vi "SMBus Block Read.vi"(5 "PEC":u8, 6 "CommandCode":u8, 7 "SlaveAddr":u8, 9 "SMBUSIndex":i32, 10 "DevIndex":i32, 11 "DevType":i32) -> (1 "function return":i32, 2 "pByteCount":u8, 3 "pData":u8[](array[numeric]))   [LabVIEW 2010, in "ControlSMBus.lvlib"]
doc: "int WINAPI SMBus_BlockRead(int DevType,int DevIndex,int SMBUSIndex,unsigned char SlaveAddr,unsigned char CommandCode,unsigned char *pData,unsigned char *pByteCount,unsigned char PEC);"
uses:
  ControlSMBus.lvlib
  ControlSMBus/Ginkgo_Driver.dll
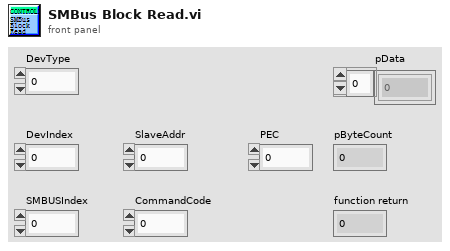
[diagram p1: front panel]
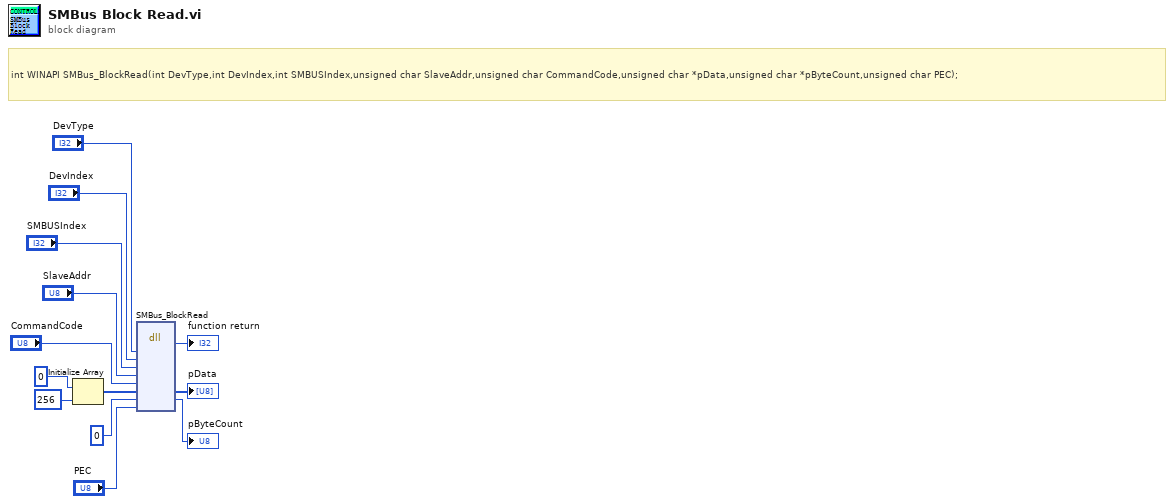
[diagram p0: block diagram]
diagram:
  # "int WINAPI SMBus_BlockRead(int DevType,int DevIndex,int SMBUSIndex,unsigned char SlaveAddr,unsigned char CommandCode,unsigned char *pData,unsigned char *pByteCount,unsigned char PEC);"
  n1 = Initialize Array(u8 0 ("element"), 256 ("dimension size")) -> (w7:u8[])
  n2 = dll-call lib="E:/Project/vt_ginkgo/truck/Ginkgo Driver/vs2010/Ginkgo_USB-I2C&SPI&CAN_API_v2.0.3.3/lib/labview_32bit/ControlSMBus/Ginkgo_Driver.*" fn="SMBus_BlockRead"("DevType"="DevType", "DevIndex"="DevIndex", "SMBUSIndex"="SMBUSIndex", "SlaveAddr"="SlaveAddr", "CommandCode"="CommandCode", "pData"=w7, "pByteCount"=u8 0, "PEC"="PEC") -> (→"function return":i32, "pData"=→"pData":u8[], "pByteCount"=→"pByteCount":u8)  [unwired: 9 in, 2 out]
